vi "X509_store_get_value_by_index.vi"(8 "error in (no error)":errorcluster, 10 "Index":i32, 11 "SSL-Context in":refnum<class "SSL-Context.lvclass">) -> (0 "error out":errorcluster, 2 "X509 cert out":refnum<class "X509-Cert.lvclass">, 3 "SSL-Context out":refnum<class "SSL-Context.lvclass">)   [LabVIEW 2013, in "OpenSSL Socket.lvlib" / "SSL-Context.lvclass"]
uses:
  SSL-Context.lvclass
  X509-Cert/X509-Cert.lvclass
  SSL-Lib/SSL-Lib.lvclass/SSL-Lib.ctl
  X509-Cert/X509-Cert.lvclass/X509-Cert.ctl
  SSL-Lib/Read Crypto Library Path.vi
  X509-Cert/Write Handle.vi
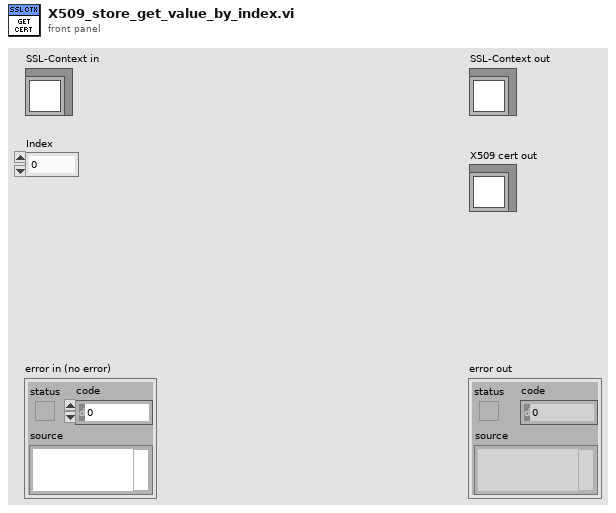
[diagram p1: front panel]
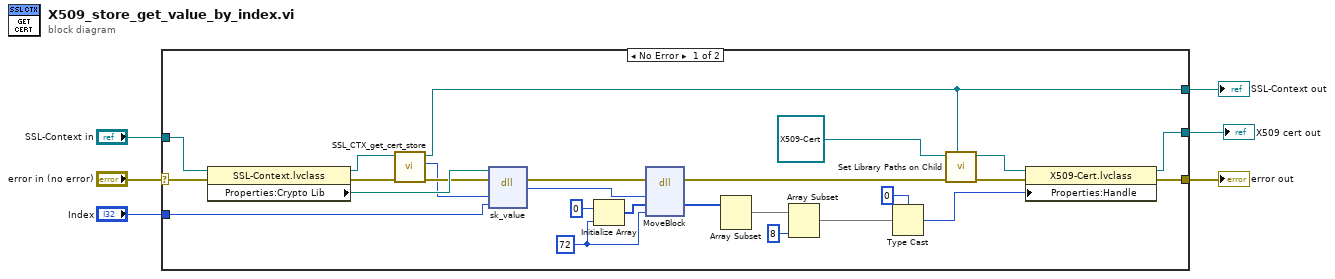
[diagram p0: block diagram]
diagram:
  n1 = case shown="No Error" "error in (no error)" {
    selector: "error in (no error)" -> [w32 w34]
    tunnel: [w23 w34] -> w5
    tunnel: [w21 w33] -> w3
    tunnel: "SSL-Context in" -> [w31 w33]
    tunnel: "Index" -> [w25 _]
    tunnel: [w19 _] -> w1
    frame No Error {
      w14 = 72 ("size")
      n2 = property class="SSL-Context.lvclass"(reference=w31, error in=w32) -> (reference out=w28:refnum<class "SSL-Context.lvclass">, error out=w29:errorcluster, "Properties:Crypto Lib"=w30:path)
      n3 = call "SSL_CTX_get_cert_store.vi"("error in (no error)"=w29, "SSL-Context in"=w28) -> ("error out"=w27:errorcluster, "X509 Cert Store"=w26:u64, "SSL-Context out"=w21:refnum<class "SSL-Context.lvclass">)  [unwired: 7 in]
      n4 = dll-call lib="C:/Program Files (x86)/National Instruments/Shared/nissl/NIlibeay32.dll" fn="sk_value"(path in=w30, error in=w27, "X509_store"=w26, "i"=w25) -> (error out=w18:errorcluster, "return type"=w17:u64)  [unwired: 3 in, 1 out]
      n5 = Initialize Array(u8 0, w14) -> (w15:u8[])
      n6 = dll-call lib="LabVIEW" fn="MoveBlock"(error in=w18, "Address"=w17, "Destination"=w15, "size"=w14) -> (error out=w7:errorcluster, "Destination"=w16:u8[])  [unwired: 5 in, 1 out]
      n7 = Array Subset(array=w16) -> (w12:u8[])  [unwired: 2 in]
      n8 = Array Subset(array=w12, length=8) -> (w10:u8[])  [unwired: 1 in]
      n9 = Type Cast(type=u64 0 ("Address"), x=w10) -> (*(type *) &x=w8:u64)
      n10 = call-dynamic "Set Library Paths on Child.vi"(7:"SSL-Lib in"=w21, "error in (no error)"=w7, 11:"SSL-Lib in"=refnum<class "X509-Cert.lvclass"> refnum ("SSL_Lib.lvlib:X509-Cert.lvclass")) -> ("error out"=w20:errorcluster, "SSL-Lib out"=w22:refnum<class "X509-Cert.lvclass">)  [unwired: 7 in]
      n11 = property class="X509-Cert.lvclass"(reference=w22, error in=w20, "Properties:Handle"=w8) -> (reference out=w19:refnum<class "X509-Cert.lvclass">, error out=w23:errorcluster)
    }
    frame Error {
    }
  }
  "error out" <- w5
  "SSL-Context out" <- w3
  "X509 cert out" <- w1
